vi "Add State(s) to Queue.vi"(0 "State(s) in Front (\"\")":string, 5 "State(s) in (\"\")":string, 7 "State(s) at Back (\"\")":string) -> (6 "States Out":string)   [LabVIEW 2013, in "JKI State Machine.lvlib"]
doc: "Concatenates states in the JKI State Machine. Unwired inputs are safely ignored and will not be added to the state queue.\n\nFor instructions on how to use the JKI State Machine, examples and video tutorials, visit:\nhttp://jkisoft.com/state-machine/\n\n<B>Inputs:</B>\n <B>State(s) in Front:</B> This allows you to place new states in the front of the state machine queue. The default is an empty string.\n <B>State(s) in:</B> Wire the existing states to this input. The default is an empty string.\n <B>State(s) in Back:</B> This allows you to place new states in the back of the state machine queue. The default is an empty string.\n\n<B>Outputs:</B>\n <B>States Out:</B>This output returns a concatenation of all the inputs seperated by a line feed character. The line feed character is required by the JKI State Machine.\n\nJKI State Machine™\nhttp://jkisoft.com/state-machine/\nCopyright (C) 2005-2008, JKI <info@jkisoft.com>\nALL RIGHTS RESERVED"
uses:
  JKI State Machine.lvlib
panel:
  # "For instructions on how to use the JKI State Machine, examples and video tutorials, visit:\nhttp://jkisoft.com/state-machine/\n\nJKI State Machine™\nhttp://jkisoft.com/state-machine/\nCopyright (C) 2005-2008, JKI <info@jkisoft.com>\nALL RIGHTS RESERVED"
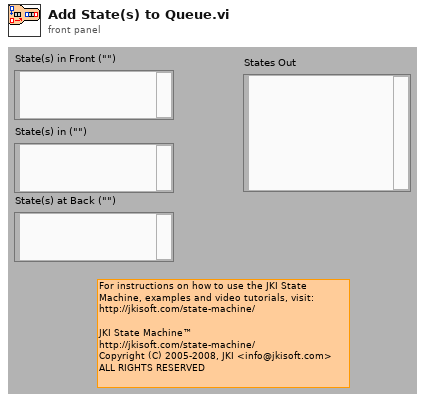
[diagram p1: front panel]
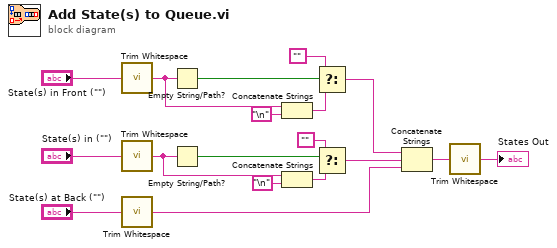
[diagram p0: block diagram]
diagram:
  n1 = call <vilib>:"Trim Whitespace.vi"("string"="State(s) in Front (\"\")") -> ("trimmed string"=w11:string)  [unwired: 1 in]
  n2 = call <vilib>:"Trim Whitespace.vi"("string"="State(s) in (\"\")") -> ("trimmed string"=w7:string)  [unwired: 1 in]
  n3 = call <vilib>:"Trim Whitespace.vi"("string"="State(s) at Back (\"\")") -> ("trimmed string"=w6:string)  [unwired: 1 in]
  n4 = Empty String/Path?(string/path=w11) -> (empty?=w15:bool)
  n5 = Empty String/Path?(string/path=w7) -> (empty?=w5:bool)
  n6 = Concatenate Strings(w11, "\n") -> (w10:string)
  n7 = Concatenate Strings(w7, "\n") -> (w8:string)
  n8 = Select(t="", s=w15, f=w10) -> (s? t:f=w14:string)
  n9 = Select(t="", s=w5, f=w8) -> (s? t:f=w13:string)
  n10 = Concatenate Strings(w14, w13, w6) -> (w2:string)
  n11 = call <vilib>:"Trim Whitespace.vi"("string"=w2) -> ("trimmed string"=→"States Out":string)  [unwired: 1 in]
